vi "未命名 2 (子VI).vi"(11 "添加的数组":refnum<vi>[](array[refnum])) -> ()   [LabVIEW 2017]
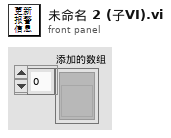
[diagram p1: front panel]
types:
  T1 = typedef "Component Assemble Input.ctl" = cluster{"Component Name":string, "Component State":bool, "D Value":i32}
  T2 = typedef "MX操作选项.ctl" = enum16{"MX Initial ", "MX Close", "X&Y&M Read", "X&Y&M Write", "D Read", "D Write", "Many component Read", "Many component Write", "Load Function Global"}
  T3 = cluster{"%Y_%m_%d_%H_%M_%S%3u":string, "%Y_%m_%d":string, "%H_%M_%S%3u":string}
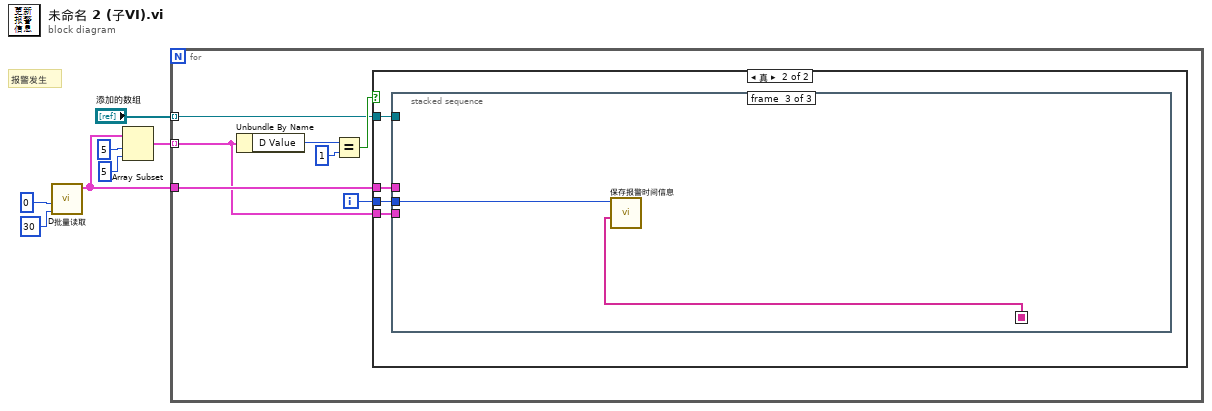
[diagram p0: block diagram]
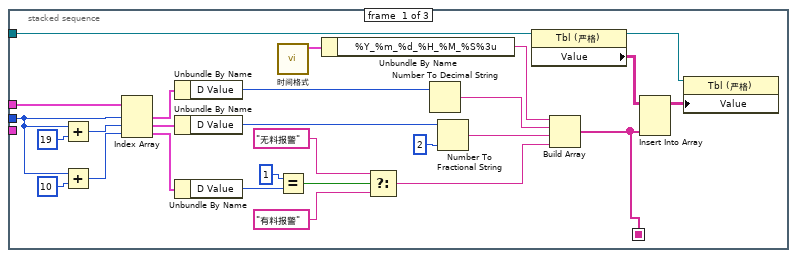
[diagram p3: hidden frame]
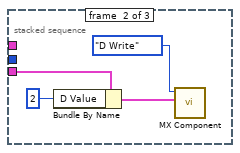
[diagram p4: hidden frame]
diagram:
  # "报警发生"
  n1 = call "D批量读取.vi"("长度"=30 ("数值"), "开始"=0) -> ("D读取"=w2:T1[])  [unwired: 9 in]
  n2 = Array Subset(array=w2, index=5 ("索引"), length=5 ("长度")) -> (w3:T1[])
  n3 = for {
    tunnel: w3 -> [w8] mode=indexing
    tunnel: w2 -> [w11]
    tunnel: "添加的数组" -> [w9] mode=indexing
    i -> [w10]
    n4 = Unbundle By Name(w8) -> ("D Value"=w14:i32)
    n5 = Equal?(x=w14, y=1) -> (x = y?=w12:bool)
    n6 = case shown="真" w12 {
      tunnel: w11 -> [_ w18]
      tunnel: w10 -> [_ w17]
      tunnel: w9 -> [_ w16]
      tunnel: w8 -> [_ w15]
      frame False {
      }
      frame True {
        n7 = stacked-sequence {
          seq-local: [w19 _ _] -> [_ _ w50]
          tunnel: w18 -> [w45 _ _]
          tunnel: w17 -> [w42 _ w51]
          tunnel: w16 -> [w28 _ _]
          tunnel: w15 -> [_ w48 _]
          frame #0 {
            n8 = Add(x=w42, y=19) -> (x+y=w43:i32)
            n9 = Add(x=w42, y=10) -> (x+y=w40:i32)
            n10 = Index Array(array=w45, index #1=w42, index #2=w43, index #3=w40) -> (element #1=w37:T1, element #2=w36:T1, element #3=w35:T1)
            n11 = Unbundle By Name(w37) -> ("D Value"=w34:i32)
            n12 = Unbundle By Name(w36) -> ("D Value"=w31:i32)
            n13 = Unbundle By Name(w35) -> ("D Value"=w32:i32)
            n14 = call "时间格式.vi"() -> ("时间格式"=w39:T3)  [unwired: 11 in]
            n15 = Equal?(x=1, y=w32) -> (x = y?=w24:bool)
            n16 = Unbundle By Name(w39) -> ("%Y_%m_%d_%H_%M_%S%3u"=w38:string)
            n17 = Select(t="无料报警", s=w24, f="有料报警") -> (s? t:f=w22:string)
            n18 = Number To Decimal String(number=w34) -> (decimal integer string=w33:string)  [unwired: 1 in]
            n19 = Number To Fractional String(number=w31, precision (6)=i16 2 ("精度(6)")) -> (F-format string=w30:string)  [unwired: 2 in]
            n20 = property class="Tbl (严格)"(reference=w28) -> (reference out=w26:refnum<vi>, "Value"=w25:string[][])  [unwired: 1 in, 1 out]
            n21 = Build Array(w38, w33, w30, w22) -> (w19:string[])
            n22 = Insert Into Array(array=w25, new element=w19) -> (w27:string[][])  [unwired: 2 in]
            n23 = property class="Tbl (严格)"(reference=w26, "Value"=w27) -> ()  [unwired: 1 in, 2 out]
          }
          frame #1 {
            n24 = Bundle By Name(cluster=w48, "D Value"=2) -> (w46:T1)
            n25 = call "MX Component.vi"("Component Assemble Input"=w46, "MX操作选项"=MX操作选项."D Write") -> ()  [unwired: 7 in, 3 out]
          }
          frame #2 {
            n26 = call "保存报警时间信息.vi"("InsertData"=w50, "设备编号"=w51) -> ()  [unwired: 10 in]
          }
        }
      }
    }
  }
